vi "Feedback Notifier.vi"(8 "error in (no error)":errorcluster, 11 "Action":enum16{"Create", "Get", "Destroy"}(ring)=enum."Destroy") -> (0 "error out":errorcluster, 3 "notifier out":refnum<notifier>)   [LabVIEW 2025]
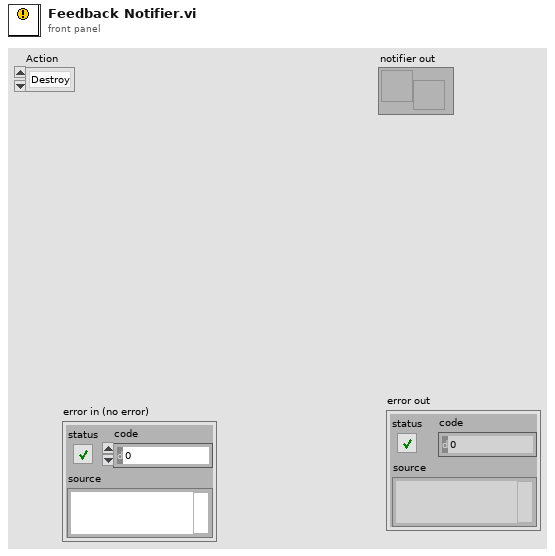
[diagram p1: front panel]
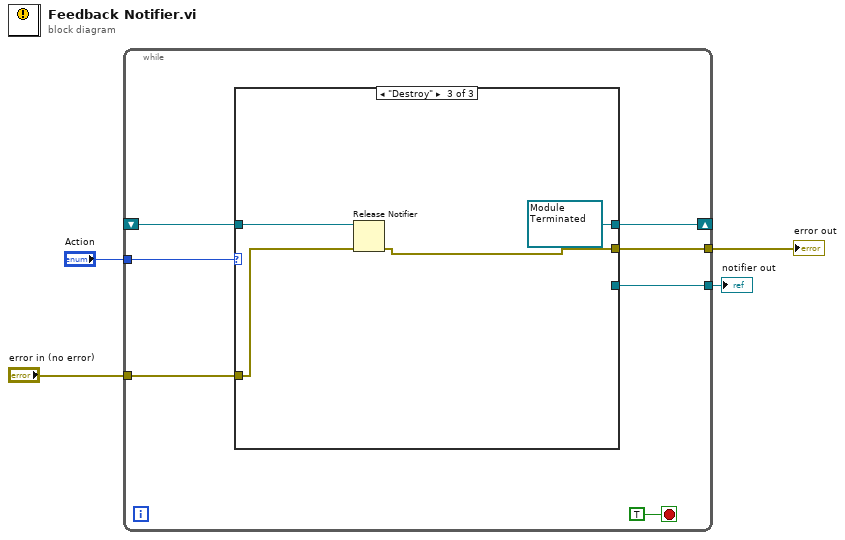
[diagram p0: block diagram]
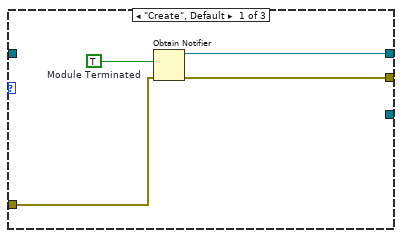
[diagram p2: hidden frame]
diagram:
  n1 = while {
    tunnel: "Action" -> [w10]
    shift-right: [w9] -> _
    shift-left: _ -> [w8]
    tunnel: "error in (no error)" -> [w7]
    tunnel: [w6] -> w2
    tunnel: [w5] -> w1
    stop <- TRUE stop-if-true
    n2 = case shown="\"Destroy\"" w10 {
      tunnel: [w15 w16 refnum<notifier> refnum ("notifier out")] -> w9
      tunnel: w8 -> [_ w16 w21]
      tunnel: w7 -> [w14 w17 w19]
      tunnel: [w13 w17 w20] -> w6
      tunnel: [_ w16 _] -> w5
      frame "Create", Default {
        w12 = TRUE  # Module Terminated
        n3 = Obtain Notifier(notification data type=w12, error in (no error)=w14) -> (notifier out=w15:refnum<notifier>, error out=w13:errorcluster)  [unwired: 2 in, 1 out]
      }
      frame "Get" {
      }
      frame "Destroy" {
        n4 = Release Notifier(notifier=w21, error in (no error)=w19) -> (error out=w20:errorcluster)  [unwired: 1 in, 2 out]
      }
    }
  }
  "error out" <- w2
  "notifier out" <- w1
